vi "MICSD Status String.vi"(8 "error in (no error)":errorcluster, 11 "VISA Resource Name":refnum<visa-resource-name>) -> (0 "error out":errorcluster, 2 "Response":string, 3 "dup VISA Resource Name":refnum<visa-resource-name>)   [LabVIEW 2020]
uses:
  <vilib>/Instr/_visa.llb/VISA Configure Serial Port (Instr).vi
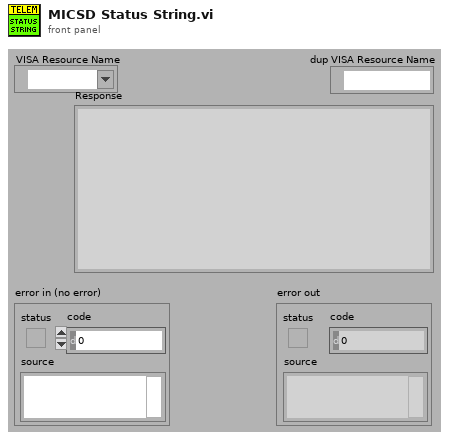
[diagram p1: front panel]
types:
  T1 = enum16{"Get Device Type", "Get Device Name", "Get Device Version", "Get Device Error"}
  T2 = cluster{"ERROR_OCCURRED":bool, "LINK_STAT_CHANGED":bool, "LINK_QUAL_CHANGED":bool, "400MHZ_TX_ACTIVE":bool, "400MHZ_RX_ACTIVE":bool, "245GHZ_TX_ACTIVE":bool, "DATA_STAT_CHANGED":bool, "SLEEPING":bool, "IDLE":bool, "SEARCHING_FOR_IMPLANT":bool, "STARTING_SESSION":bool, "LISTENING_FOR_EMERG":bool, "IN_SESSION":bool}
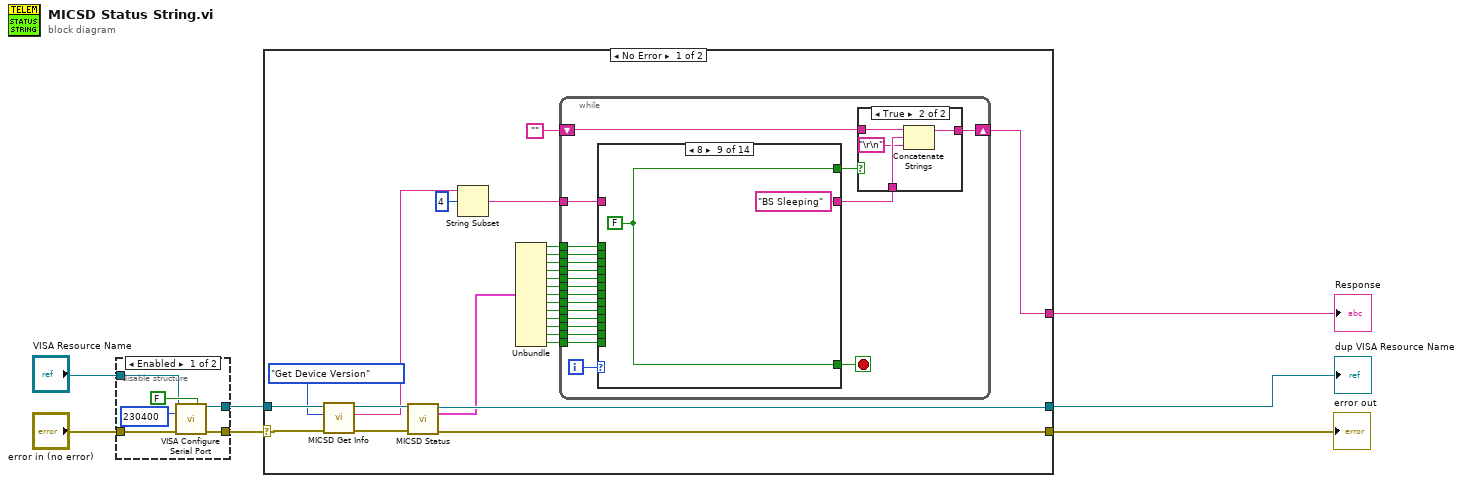
[diagram p0: block diagram]
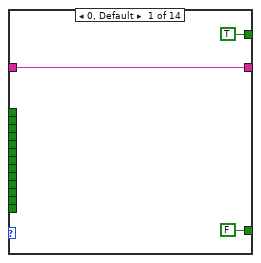
[diagram p4: hidden frame]
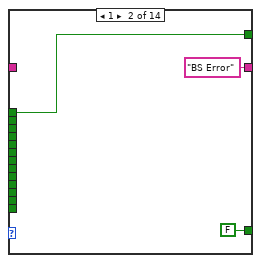
[diagram p5: hidden frame]
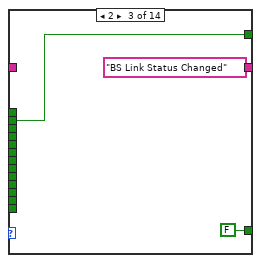
[diagram p6: hidden frame]
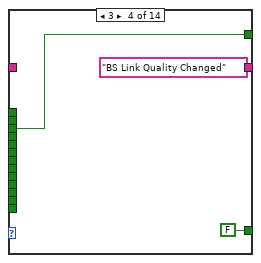
[diagram p7: hidden frame]
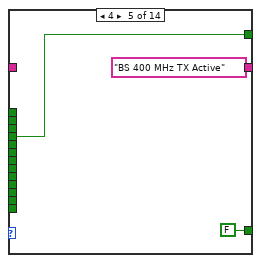
[diagram p8: hidden frame]
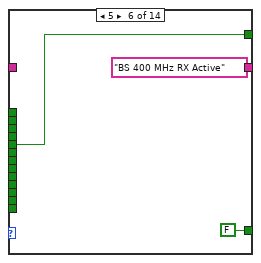
[diagram p9: hidden frame]
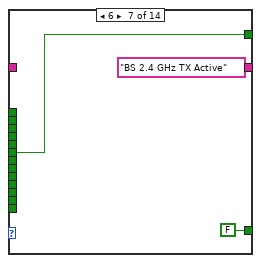
[diagram p10: hidden frame]
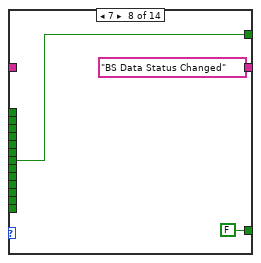
[diagram p11: hidden frame]
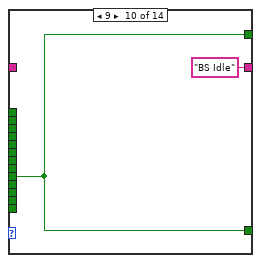
[diagram p12: hidden frame]
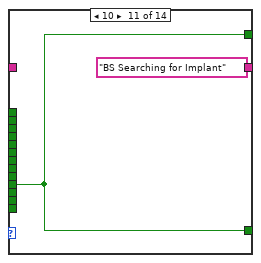
[diagram p13: hidden frame]
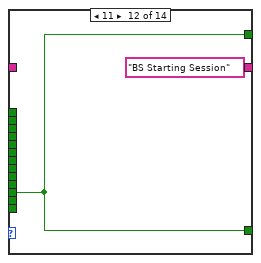
[diagram p14: hidden frame]
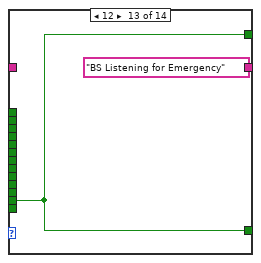
[diagram p15: hidden frame]
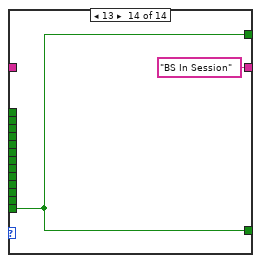
[diagram p16: hidden frame]
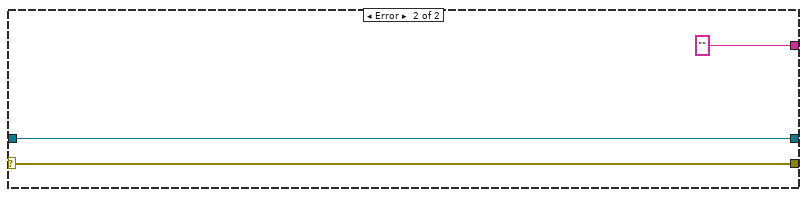
[diagram p17: hidden frame]
diagram:
  n1 = disable-structure shown="Enabled" {
    disable-tunnel: [w11 w14] -> w6
    disable-tunnel: "error in (no error)" -> [w10 w14]
    disable-tunnel: "VISA Resource Name" -> [w9 w15]
    disable-tunnel: [w8 w15] -> w3
    frame Enabled {
      n2 = call-poly "VISA Configure Serial Port"("VISA resource name"=w9, "Enable Termination\nChar (T)"=FALSE ("Enable Termination\nChar (T)"), "baud rate (9600)"=u32 230400, "error in (no error)"=w10) -> ("VISA resource name out"=w8:refnum<visa-resource-name>, "error out"=w11:errorcluster)  [unwired: 10 in]
    }
    frame Disabled {
    }
  }
  n3 = case shown="No Error" w6 {
    selector: w6 -> [w34 w105]
    tunnel: [w40 w105] -> w1
    tunnel: w3 -> [w35 w104]
    tunnel: [w41 w104] -> w7
    tunnel: [w38 "" ("type")] -> w2
    frame No Error {
      n4 = call "MICSD Get Info.vi"("error in (no error)"=w34, "Command"=T1."Get Device Version", "VISA Resource Name"=w35) -> ("error out"=w33:errorcluster, "Response"=w31:string, "dup VISA Resource Name"=w36:refnum<visa-resource-name>)  [unwired: 6 in]
      n5 = call "MICSD Status.vi"("VISA Resource Name"=w36, "error in (no error)"=w33) -> ("dup VISA Resource Name"=w41:refnum<visa-resource-name>, "Status Flags"=w39:T2, "error out"=w40:errorcluster)  [unwired: 7 in, 4 out]
      n6 = String Subset(string=w31, offset (0)=4) -> (substring=w29:string)  [unwired: 1 in]
      n7 = Unbundle(w39) -> ("ERROR_OCCURRED"=w28:bool, "LINK_STAT_CHANGED"=w27:bool, "LINK_QUAL_CHANGED"=w26:bool, "400MHZ_TX_ACTIVE"=w25:bool, "400MHZ_RX_ACTIVE"=w24:bool, "245GHZ_TX_ACTIVE"=w23:bool, "DATA_STAT_CHANGED"=w22:bool, "SLEEPING"=w21:bool, "IDLE"=w20:bool, "SEARCHING_FOR_IMPLANT"=w19:bool, "STARTING_SESSION"=w18:bool, "LISTENING_FOR_EMERG"=w17:bool, "IN_SESSION"=w16:bool)
      n8 = while {
        shift-right: [w45] -> w38
        shift-left: "" -> [w46]
        tunnel: w29 -> [w60]
        tunnel: w28 -> [w59]
        tunnel: w27 -> [w58]
        tunnel: w26 -> [w57]
        tunnel: w25 -> [w56]
        tunnel: w24 -> [w55]
        tunnel: w23 -> [w54]
        tunnel: w22 -> [w53]
        tunnel: w21 -> [w52]
        tunnel: w20 -> [w51]
        tunnel: w19 -> [w50]
        tunnel: w18 -> [w49]
        tunnel: w17 -> [w48]
        tunnel: w16 -> [w47]
        i -> [w61]
        stop <- w42 stop-if-true
        n9 = case shown="8" w61 {
          tunnel: w60 -> [w69 _ _ _ _ _ _ _ _ _ _ _ _ _]
          tunnel: w59 -> [_ w72 _ _ _ _ _ _ _ _ _ _ _ _]
          tunnel: w58 -> [_ _ w75 _ _ _ _ _ _ _ _ _ _ _]
          tunnel: w57 -> [_ _ _ w77 _ _ _ _ _ _ _ _ _ _]
          tunnel: w56 -> [_ _ _ _ w79 _ _ _ _ _ _ _ _ _]
          tunnel: w55 -> [_ _ _ _ _ w82 _ _ _ _ _ _ _ _]
          tunnel: w54 -> [_ _ _ _ _ _ w85 _ _ _ _ _ _ _]
          tunnel: w53 -> [_ _ _ _ _ _ _ w88 _ _ _ _ _ _]
          tunnel: w52 -> [_ _ _ _ _ _ _ _ _ _ _ _ _ _]
          tunnel: w51 -> [_ _ _ _ _ _ _ _ _ w93 _ _ _ _]
          tunnel: w50 -> [_ _ _ _ _ _ _ _ _ _ w95 _ _ _]
          tunnel: w49 -> [_ _ _ _ _ _ _ _ _ _ _ w97 _ _]
          tunnel: w48 -> [_ _ _ _ _ _ _ _ _ _ _ _ w99 _]
          tunnel: w47 -> [_ _ _ _ _ _ _ _ _ _ _ _ _ w101]
          tunnel: [w69 "BS Error" ("Response") "BS Link Status Changed" ("Response") "BS Link Quality Changed" ("Response") "BS 400 MHz TX Active" ("Response") "BS 400 MHz RX Active" ("Response") "BS 2.4 GHz TX Active" ("Response") "BS Data Status Changed" ("Response") "BS Sleeping" ("Response") "BS Idle" ("Response") "BS Searching for Implant" ("Response") "BS Starting Session" ("Response") "BS Listening for Emergency" ("Response") "BS In Session" ("Response")] -> w44
          tunnel: [TRUE ("IN_SESSION") w72 w75 w77 w79 w82 w85 w88 w91 w93 w95 w97 w99 w101] -> w43
          tunnel: [FALSE FALSE FALSE FALSE FALSE FALSE FALSE FALSE w91 w93 w95 w97 w99 w101] -> w42
          frame 0, Default {
          }
          frame 1 {
          }
          frame 2 {
          }
          frame 3 {
          }
          frame 4 {
          }
          frame 5 {
          }
          frame 6 {
          }
          frame 7 {
          }
          frame 8 {
            w91 = FALSE ("IN_SESSION")
          }
          frame 9 {
          }
          frame 10 {
          }
          frame 11 {
          }
          frame 12 {
          }
          frame 13 {
          }
        }
        n10 = case shown="True" w43 {
          tunnel: w46 -> [w62 w66]
          tunnel: [w62 w65] -> w45
          tunnel: w44 -> [_ w64]
          frame False {
          }
          frame True {
            n11 = Concatenate Strings(w66, w64, "\r\n") -> (w65:string)
          }
        }
      }
    }
    frame Error {
    }
  }
  "dup VISA Resource Name" <- w7
  "error out" <- w1
  "Response" <- w2
